vi "path-list.vi"(10 "Folder":path) -> (2 "Files":path[](array[path]))   [LabVIEW 2017]
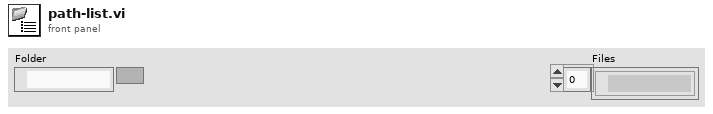
[diagram p1: front panel]
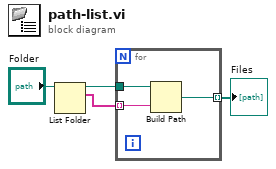
[diagram p0: block diagram]
diagram:
  n1 = List Folder(path="Folder") -> (path out=w4:path, filenames=w3:string[])  [unwired: 3 in, 2 out]
  n2 = for {
    tunnel: w4 -> [w7]
    tunnel: w3 -> [w6] mode=indexing
    tunnel: [w5] -> w2 mode=indexing
    n3 = Build Path(base path=w7, name or relative path=w6) -> (appended path=w5:path)
  }
  "Files" <- w2
